vi "Check and compute displacements.vi"(6 "x pixel displacement 2":dbl, 7 "x pixel displacement 1":dbl, 8 "error in (no error)":errorcluster, 9 "y pixel displacement 2":dbl, 10 "y pixel displacement 1":dbl, 11 "Retiga in":refnum<class "Retiga.lvclass">) -> (0 "error out":errorcluster, 1 "fine?":bool, 2 "translation out":dbl[unit], 3 "Retiga out":refnum<class "Retiga.lvclass">)   [LabVIEW 2012, in "Retiga.lvclass"]
uses:
  Retiga.lvclass
  Retiga.lvclass/Retiga.ctl
  <vilib>/addons/control/pid/pid.llb/PID (DBL).vi
  <vilib>/addons/control/pid/NI_PID_pid.lvlib
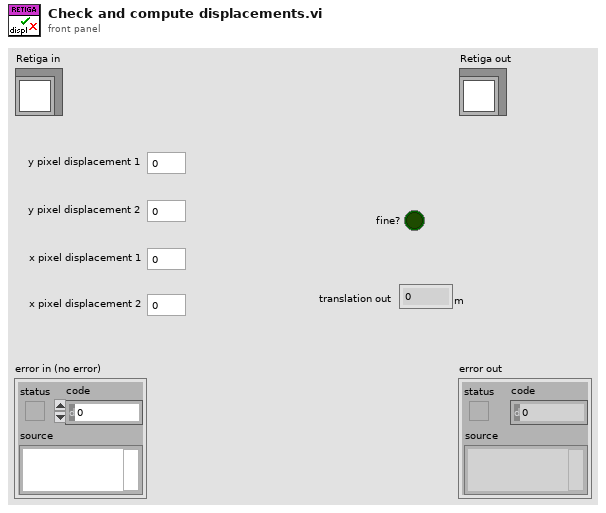
[diagram p1: front panel]
types:
  T1 = cluster{"proportional gain (Kc)":dbl, "integral time (Ti, min)":dbl, "derivative time (Td, min)":dbl}
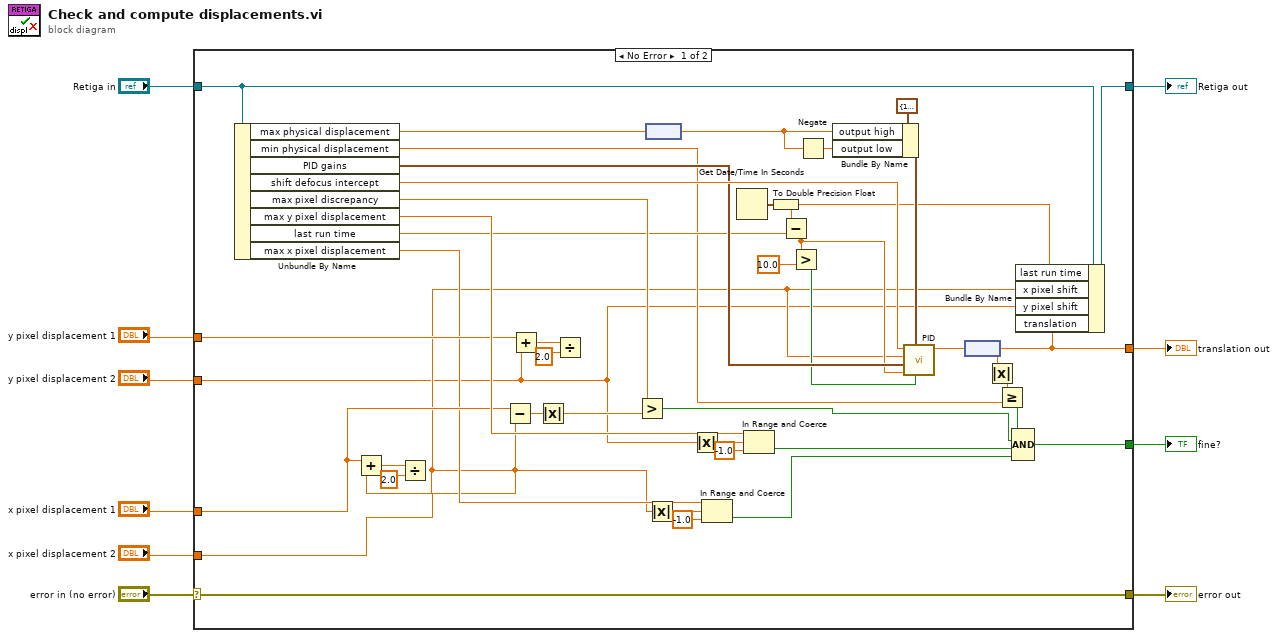
[diagram p0: block diagram]
diagram:
  n1 = case shown="No Error" "error in (no error)" {
    selector: "error in (no error)" -> [w52 w54]
    tunnel: [w52 w54] -> w9
    tunnel: [w39 w53] -> w7
    tunnel: "Retiga in" -> [w40 w53]
    tunnel: "y pixel displacement 1" -> [w38 _]
    tunnel: "y pixel displacement 2" -> [w11 _]
    tunnel: "x pixel displacement 1" -> [w35 _]
    tunnel: "x pixel displacement 2" -> [w12 _]
    tunnel: [w16 _] -> w2
    tunnel: [w37 _] -> w1
    frame No Error {
      n2 = Unbundle By Name(w40) -> ("max physical displacement"=w21:dbl[unit], "min physical displacement"=w18:dbl[unit], "PID gains"=w30:T1, "shift defocus intercept"=w31:dbl, "max pixel discrepancy"=w46:dbl, "max y pixel displacement"=w41:dbl, "last run time"=w29:dbl, "max x pixel displacement"=w33:dbl)
      n3 = Add(x=w35, y=w12) -> (x+y=w43:dbl)
      n4 = Divide(x=w43, y=2.0) -> ()  [unwired: 1 out]
      n5 = Subtract(x=w35, y=w12) -> (x-y=w50:dbl)
      n6 = Add(x=w38, y=w11) -> (x+y=w49:dbl)
      n7 = Absolute Value(x=w50) -> (abs(x)=w51:dbl)
      n8 = Divide(x=w49, y=2.0) -> ()  [unwired: 1 out]
      n9 = Greater?(x=w46, y=w51) -> (0:w13:bool)
      n10 = node(w21) -> (w19:dbl)
      n11 = Absolute Value(x=w12) -> (abs(x)=w36:dbl)
      n12 = Absolute Value(x=w11) -> (abs(x)=w42:dbl)
      n13 = In Range and Coerce(upper limit=w33, x=w36, lower limit=-1.0) -> (In Range?=w45:bool)  [unwired: 1 out]
      n14 = Get Date/Time In Seconds() -> (seconds since 1Jan1904=w28:timestamp)
      n15 = In Range and Coerce(upper limit=w41, x=w42, lower limit=-1.0) -> (In Range?=w47:bool)  [unwired: 1 out]
      n16 = To Double Precision Float(number=w28) -> (double precision float=w14:dbl)
      n17 = Subtract(x=w14, y=w29) -> (x-y=w26:dbl)
      n18 = Greater?(x=w26, y=10.0) -> (0:w25:bool)
      n19 = Negate(x=w19) -> (-x=w20:dbl)
      n20 = Bundle By Name(cluster=cluster{"output high":dbl, "output low":dbl} {"output high"=100.0, "output low"=-100.0} ("output range"), "output high"=w19, "output low"=w20) -> (w22:cluster{"output high":dbl, "output low":dbl})
      n21 = call-poly <vilib>:"PID.vi"("reinitialize? (F)"=w25, "output range"=w22, "dt (s)"=w26, "PID gains"=w30, "process variable"=w12, "setpoint"=w31) -> ("output"=w24:dbl)  [unwired: 4 in, 1 out]
      n22 = node(w24) -> (w16:dbl[unit])
      n23 = Absolute Value(x=w16) -> (abs(x)=w17:dbl[unit])
      n24 = Greater Or Equal?(x=w17, y=w18) -> (x >= y?=w15:bool)
      n25 = Compound Arithmetic op=AND(w15, w13, w47, w45) -> (w37:bool)
      n26 = Bundle By Name(cluster=w40, "last run time"=w14, "x pixel shift"=w12, "y pixel shift"=w11, "translation"=w16) -> (w39:refnum<class "Retiga.lvclass">)
    }
    frame Error {
    }
  }
  "error out" <- w9
  "Retiga out" <- w7
  "fine?" <- w1
  "translation out" <- w2
